vi "DriveForDistance.vi"() -> ()   [LabVIEW 2018]
uses:
  Framework/Robot Global Data.vi
  Drive/Implementation/Drive Published Globals.vi
panel:
  in  "NoWait":bool
  in  "Speed":dbl
  in  "Distance":dbl
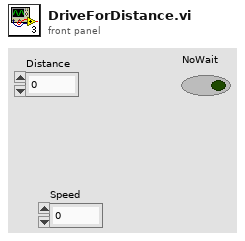
[diagram p1: front panel]
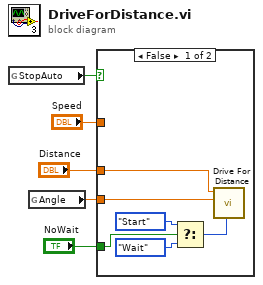
[diagram p0: block diagram]
diagram:
  n1 = global read "Robot Global Data.vi" "StopAuto"() -> (w2:bool)
  n2 = global read "Drive Published Globals.vi" "Angle"() -> (w1:dbl)
  n3 = case shown="False" w2 {
    tunnel: "Distance" -> [w7 _]
    tunnel: "Speed" -> [_ _]
    tunnel: "NoWait" -> [w9 _]
    tunnel: w1 -> [w6 _]
    frame False {
      n4 = Select(t=enum16{"Start", "Wait"}."Start" ("Synchronization"), s=w9, f=enum16{"Start", "Wait"}."Wait" ("Synchronization")) -> (s? t:f=w8:enum16{"Start", "Wait"})
      n5 = call "Drive For Distance.vi"("Synchronication"=w8, "Angle"=w6, "Distance"=w7) -> ()  [unwired: 8 in, 1 out]
    }
    frame True {
    }
  }
